vi "kinfe edge method.vi"(0 "Speed":cluster{"Speed":i32, "Vi":i32, "Vi steps":i32}={"Speed"=8000, "Vi"=1000, "Vi steps"=800} {"Speed" min=50 max=8000 step=50 scale=50.0..8000.0}, 1 "Go_stop":bool, 2 "PosCtrl":T5={"Go x"=FALSE, "Back x"=FALSE, "Go y"=FALSE, "Back y"=FALSE, "Go z"=FALSE, "Back z"=FALSE, "dX (um)"=1000, "dY (um)"=0, "dZ (um)"=0} {"dX (um)" step=1}, 5 "Home":bool, 7 "Zero":bool, 10 "stop 2":bool, 11 "VISA resource (RS232)":refnum<visa-resource-name>="COM1") -> (3 "?":cluster{"X":dbl, "Y":dbl, "Z":dbl}, 9 "Static":bool)   [LabVIEW 2018]
uses:
  <vilib>/userdefined/High Color/IMAQdx.ctl
  <vilib>/Instr/_visa.llb/VISA Configure Serial Port (Instr).vi
  <vilib>/vision/driver/NI_Vision_Acquisition_Software.lvlib
panel:
  out "t&Y error":dbl[][](array[numeric])
  out "um/s":string
  out "um(x) 2":string
  out "um(y)":string
  out "appended array":dbl[](array[numeric])
  out "fitting (y&T)":dbl[][](array[numeric])
  out "path (for logistic)":path
  out "row data save path":path
  in  "cluster":cluster{"T&Y(output)":dbl[][], "dt":dbl} {"dt" format="%#_13g"}
  out "T&Y(output)":dbl[][](array[numeric])
  out "Y(output)":dbl[](array[numeric])
  out "T(output)":dbl[](array[numeric])
  out "Initial X":dbl format="%^.3e"
  out "X Increment":dbl format="%^.3e"
  out "Y(all)":dbl[](array[numeric]) caption="Waveform Array" format="%^.3e"
  out "T(all)":dbl[](array[numeric])
  in  "Tout":i32
  in  "timeout":i32=5000 caption="Timeout\n[ms]"
  out "Waveform":T1(graph)
  out "Acquisitions":i32
  in  "Tab Control 2":enum32{"knife edge method", "Setting"}(tab)
  out "Snap Image":T2(plugin-control)
  in  "Get Image":bool
  in  "Tab Control":enum32{"Error function", "logistic function"}(tab)
  out "fitting":cluster{cdb[]}[](graph)
  in  "Paramter guess 2":dbl[](array[numeric])=[165.0, 0.2, 0.1]
  out "best fit parameters":dbl[](array[numeric])
  out "x0":dbl
  out "c":dbl
  in  "index":i32
  out "middle index(es)":i32
  out "number of function calls":i32
  in  "fitting(error)":bool caption="Fitting"
  in  "save(error)":bool caption="Fitting"
  in  "save(Logistic)":bool caption="Fitting"
  in  "fitting(Logistic)":bool caption="Fitting"
  out "output cluster 2":T3
  in  "Paramter guess":dbl[](array[numeric])=[-4.2, 0.0, 100.0, 1.0, 1.0]
  out "E":i32
  out "XY Graph":cluster{cdb[]}[](graph)
  out "output cluster":T4
  in  "speed(um/s)":i32
  in  "move(um)":i32
  in  "knife edge method":bool caption="Start"
  in  "knife edge method(stop)":bool caption="Start"
  in  "Tab Control 3":enum32{"read 2", "read", "cut & save"}(tab)
  in  "?":enum32{" RS232", "ESP32"}(tab)
  in  "x-":bool caption="Start"
  in  "x+":bool caption="Start"
  out "um(x)":string
  in  "y+":bool caption="Start"
  in  "y-":bool caption="Start"
  in  "um":i32
  in  "um":i32
  in  "channel on":i32=1 min=1 max=4 step=1
  out "ActiveChannels":i32[](array[numeric])=[1, 4]
  in  "Start":bool
  in  "Single":bool
  in  "Stop":bool
  in  "Exit":bool
  out "Samples count":i32[](array[numeric])
  out "waveform 3":cluster{"T":dbl[], "Waveform Array":dbl[]}(graph)
  out "point":i32
  in  "Path":path
  in  "name":string
  in  "Slide":cluster{dbl, dbl}(slide)={0.0, 1.2121212121212122} scale=0.10601..1.1059999999987864
  in  "Save data":bool caption="Fitting"
  out "waveform 2":cluster{"T":dbl[], "Waveform Array":dbl[]}(graph)
  out "Grab Image":T2(plugin-control)
  in  "?":bool
  in  "VISA resource name 2":refnum<visa-resource-name>="TCPIP0::169.254.236.131::inst0::INSTR" caption="VISA resource name"
  in  "VISA resource name":refnum<visa-resource-name>="TCPIP::169.254.236.131::HISLIP"
  out "Moving Time (Sec)":dbl
  in  "VISA resource (esp32)":refnum<visa-resource-name>="COM8"
  in  "Delay (ms)":u32=100
  in  "update period (ms)":u32=100
  in  "Go":bool
  in  "Back":bool
  in  "X0":T6 {"Y (um)" min=0.0; "X (um)" min=0.0}
  in  "Scaling":cluster{"X":u16, "Y":u16, "Z":u16} {"Z" items=["X", "Z", "None"]; "Y" items=["X", "Z", "None"]; "X" items=["X", "Z", "None"]}
  in  "Position to go":T7={"Position"={"X"=FALSE, "Target X (um)"=1000.0, "Current X (um)"=1000.0, "Scaling X"=0, "Y"=FALSE, "Target Y (um)"=0.0, "Current Y (um)"=0.0, "Scaling Y"=0, "Z"=FALSE, "Target Z (um)"=0.0, "Current Z (um)"=0.0, "Scaling Z"=0}, "Speed"={"Speed"=3111, "Vi steps"=800, "Vi"=1000}} {"Speed"."Speed" min=50 max=8000 step=50 scale=50.0..8000.0; "Position"."Current X (um)" step=1.0; "Position"."Scaling Z" items=["X", "Z", "None"]; "Position"."Scaling Y" items=["X", "Z", "None"]; "Position"."Scaling X" items=["X", "Z", "None"]; "Position"."Target X (um)" step=1.0}
  in  "Camera COM":T8
  out "Position Info":T9={"Current coordinates"={"Steps"=0.0, "X"=FALSE, "Steps 2"=0.0, "Y"=FALSE, "Steps 3"=0.0, "Z"=FALSE}, "read buffer"="", "Command"="a", "Current coordinates 2"={"X"=0.0, "Y"=0.0, "Z"=0.0}, "Moving Time (Sec)"=0.0}
  out "RS232 error":errorcluster
  # "Only For Knife Edge Method"
  # "y0\n\nx0\n\nK\n\nL\n\nA"
  # "Esp32"
  # "CCD"
  # "RTO"
  # "RS232"
  # "Origin"
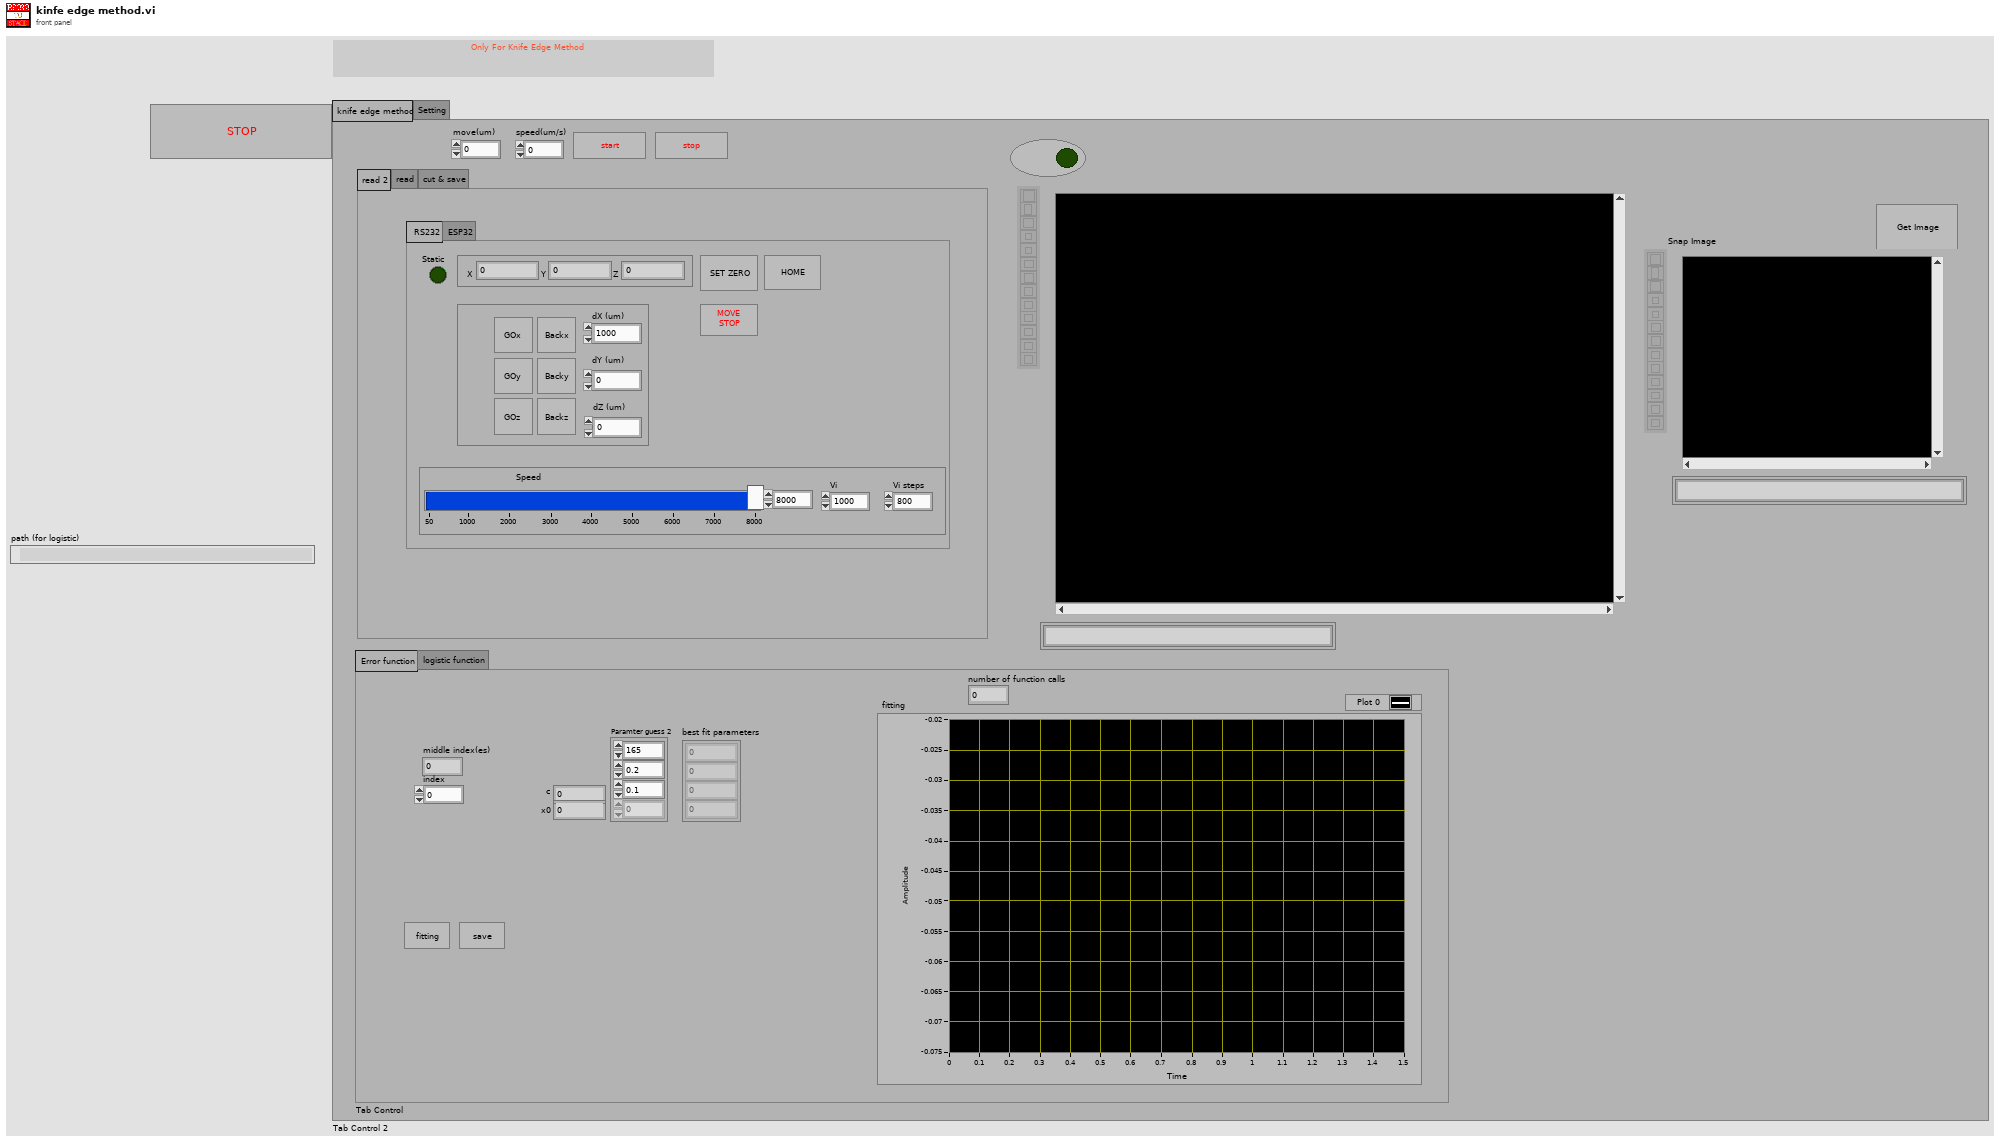
[diagram p1: front panel]
types:
  T1 = cluster{"Initial X":dbl, "X Increment":dbl, "Waveform Array":dbl[]}[]
  T2 = typedef "IMAQ Image.ctl" = refnum<image>
  T3 = cluster{"y0":dbl, "x0":dbl, "best fit parameters":dbl[]}
  T4 = cluster{"T(all)":dbl[], "Y(all)":dbl[], "X Increment":dbl, "Initial X":dbl}
  T5 = cluster{"Go x":bool, "Back x":bool, "Go y":bool, "Back y":bool, "Go z":bool, "Back z":bool, "dX (um)":u32, "dY (um)":u32, "dZ (um)":u32}
  T6 = cluster{"X (um)":dbl, "X 2":bool, "Y (um)":dbl, "Y 2":bool, "Z (um)":dbl, "Z 2":bool}
  T7 = cluster{"Position":cluster{"X":bool, "Target X (um)":dbl, "Current X (um)":dbl, "Scaling X":u16, "Y":bool, "Target Y (um)":dbl, "Current Y (um)":dbl, "Scaling Y":u16, "Z":bool, "Target Z (um)":dbl, "Current Z (um)":dbl, "Scaling Z":u16}, "Speed":cluster{"Speed":i32, "Vi steps":i32, "Vi":i32}}
  T8 = typedef "IMAQdx.ctl" = refnum<k21>
  T9 = cluster{"Current coordinates":cluster{"Steps":dbl, "X":bool, "Steps 2":dbl, "Y":bool, "Steps 3":dbl, "Z":bool}, "read buffer":string, "Command":string, "Current coordinates 2":cluster{"X":dbl, "Y":dbl, "Z":dbl}, "Moving Time (Sec)":dbl}
  T10 = cluster{"X":bool, "Target X (um)":dbl, "Current X (um)":dbl, "Scaling X":u16, "Y":bool, "Target Y (um)":dbl, "Current Y (um)":dbl, "Scaling Y":u16, "Z":bool, "Target Z (um)":dbl, "Current Z (um)":dbl, "Scaling Z":u16}
  T11 = cluster{"Go x":bool, "Back x":bool, "Go y":bool, "Back y":bool, "Go z":bool, "Back z":bool, "dX (um)":dbl, "dY (um)":dbl, "dZ (um)":dbl}
  T12 = cluster{"Position":cluster{"X":bool, "Target X (um)":dbl, "Current X (um)":dbl, "Scaling X":u16, "Y":bool, "Target Y (um)":dbl, "Current Y (um)":dbl, "Scaling Y":u16, "Z":bool, "Target Z (um)":dbl, "Current Z (um)":dbl, "Scaling Z":u16}, "Value":cluster{"Speed":i32, "Vi":i32, "Vi steps":i32}}
  T13 = cluster{"Task":u16, cluster{"Position":cluster{"X":bool, "Target X (um)":dbl, "Current X (um)":dbl, "Scaling X":u16, "Y":bool, "Target Y (um)":dbl, "Current Y (um)":dbl, "Scaling Y":u16, "Z":bool, "Target Z (um)":dbl, "Current Z (um)":dbl, "Scaling Z":u16}, "Value":cluster{"Speed":i32, "Vi":i32, "Vi steps":i32}}}
  T14 = cluster{"Task":u16, "Position to go":cluster{"Position":cluster{"X":bool, "Target X (um)":dbl, "Current X (um)":dbl, "Scaling X":u16, "Y":bool, "Target Y (um)":dbl, "Current Y (um)":dbl, "Scaling Y":u16, "Z":bool, "Target Z (um)":dbl, "Current Z (um)":dbl, "Scaling Z":u16}, "Speed":cluster{"Speed":i32, "Vi steps":i32, "Vi":i32}}}
  T15 = cluster{"Task 2":u16, "Position to go 2":cluster{"Position":cluster{"X":bool, "Target X (um)":dbl, "Current X (um)":dbl, "Scaling X":u16, "Y":bool, "Target Y (um)":dbl, "Current Y (um)":dbl, "Scaling Y":u16, "Z":bool, "Target Z (um)":dbl, "Current Z (um)":dbl, "Scaling Z":u16}, "Speed":cluster{"Speed":i32, "Vi steps":i32, "Vi":i32}}}
  T16 = cluster{"Go x":bool, "Back x":bool, "Go y":bool, "Back y":bool, "Go z":bool, "Back z":bool, "dX (um)":bool, "dY (um)":bool, "dZ (um)":bool}
  T17 = cluster{"Initial X":dbl, "X Increment":dbl, "Waveform Array":dbl[]}
  T18 = cluster{"Ring":u16, "Value":cluster{"Position":cluster{"X":bool, "Target X (um)":dbl, "Current X (um)":dbl, "Scaling X":u16, "Y":bool, "Target Y (um)":dbl, "Current Y (um)":dbl, "Scaling Y":u16, "Z":bool, "Target Z (um)":dbl, "Current Z (um)":dbl, "Scaling Z":u16}, "Speed":cluster{"Speed":i32, "Vi steps":i32, "Vi":i32}}}
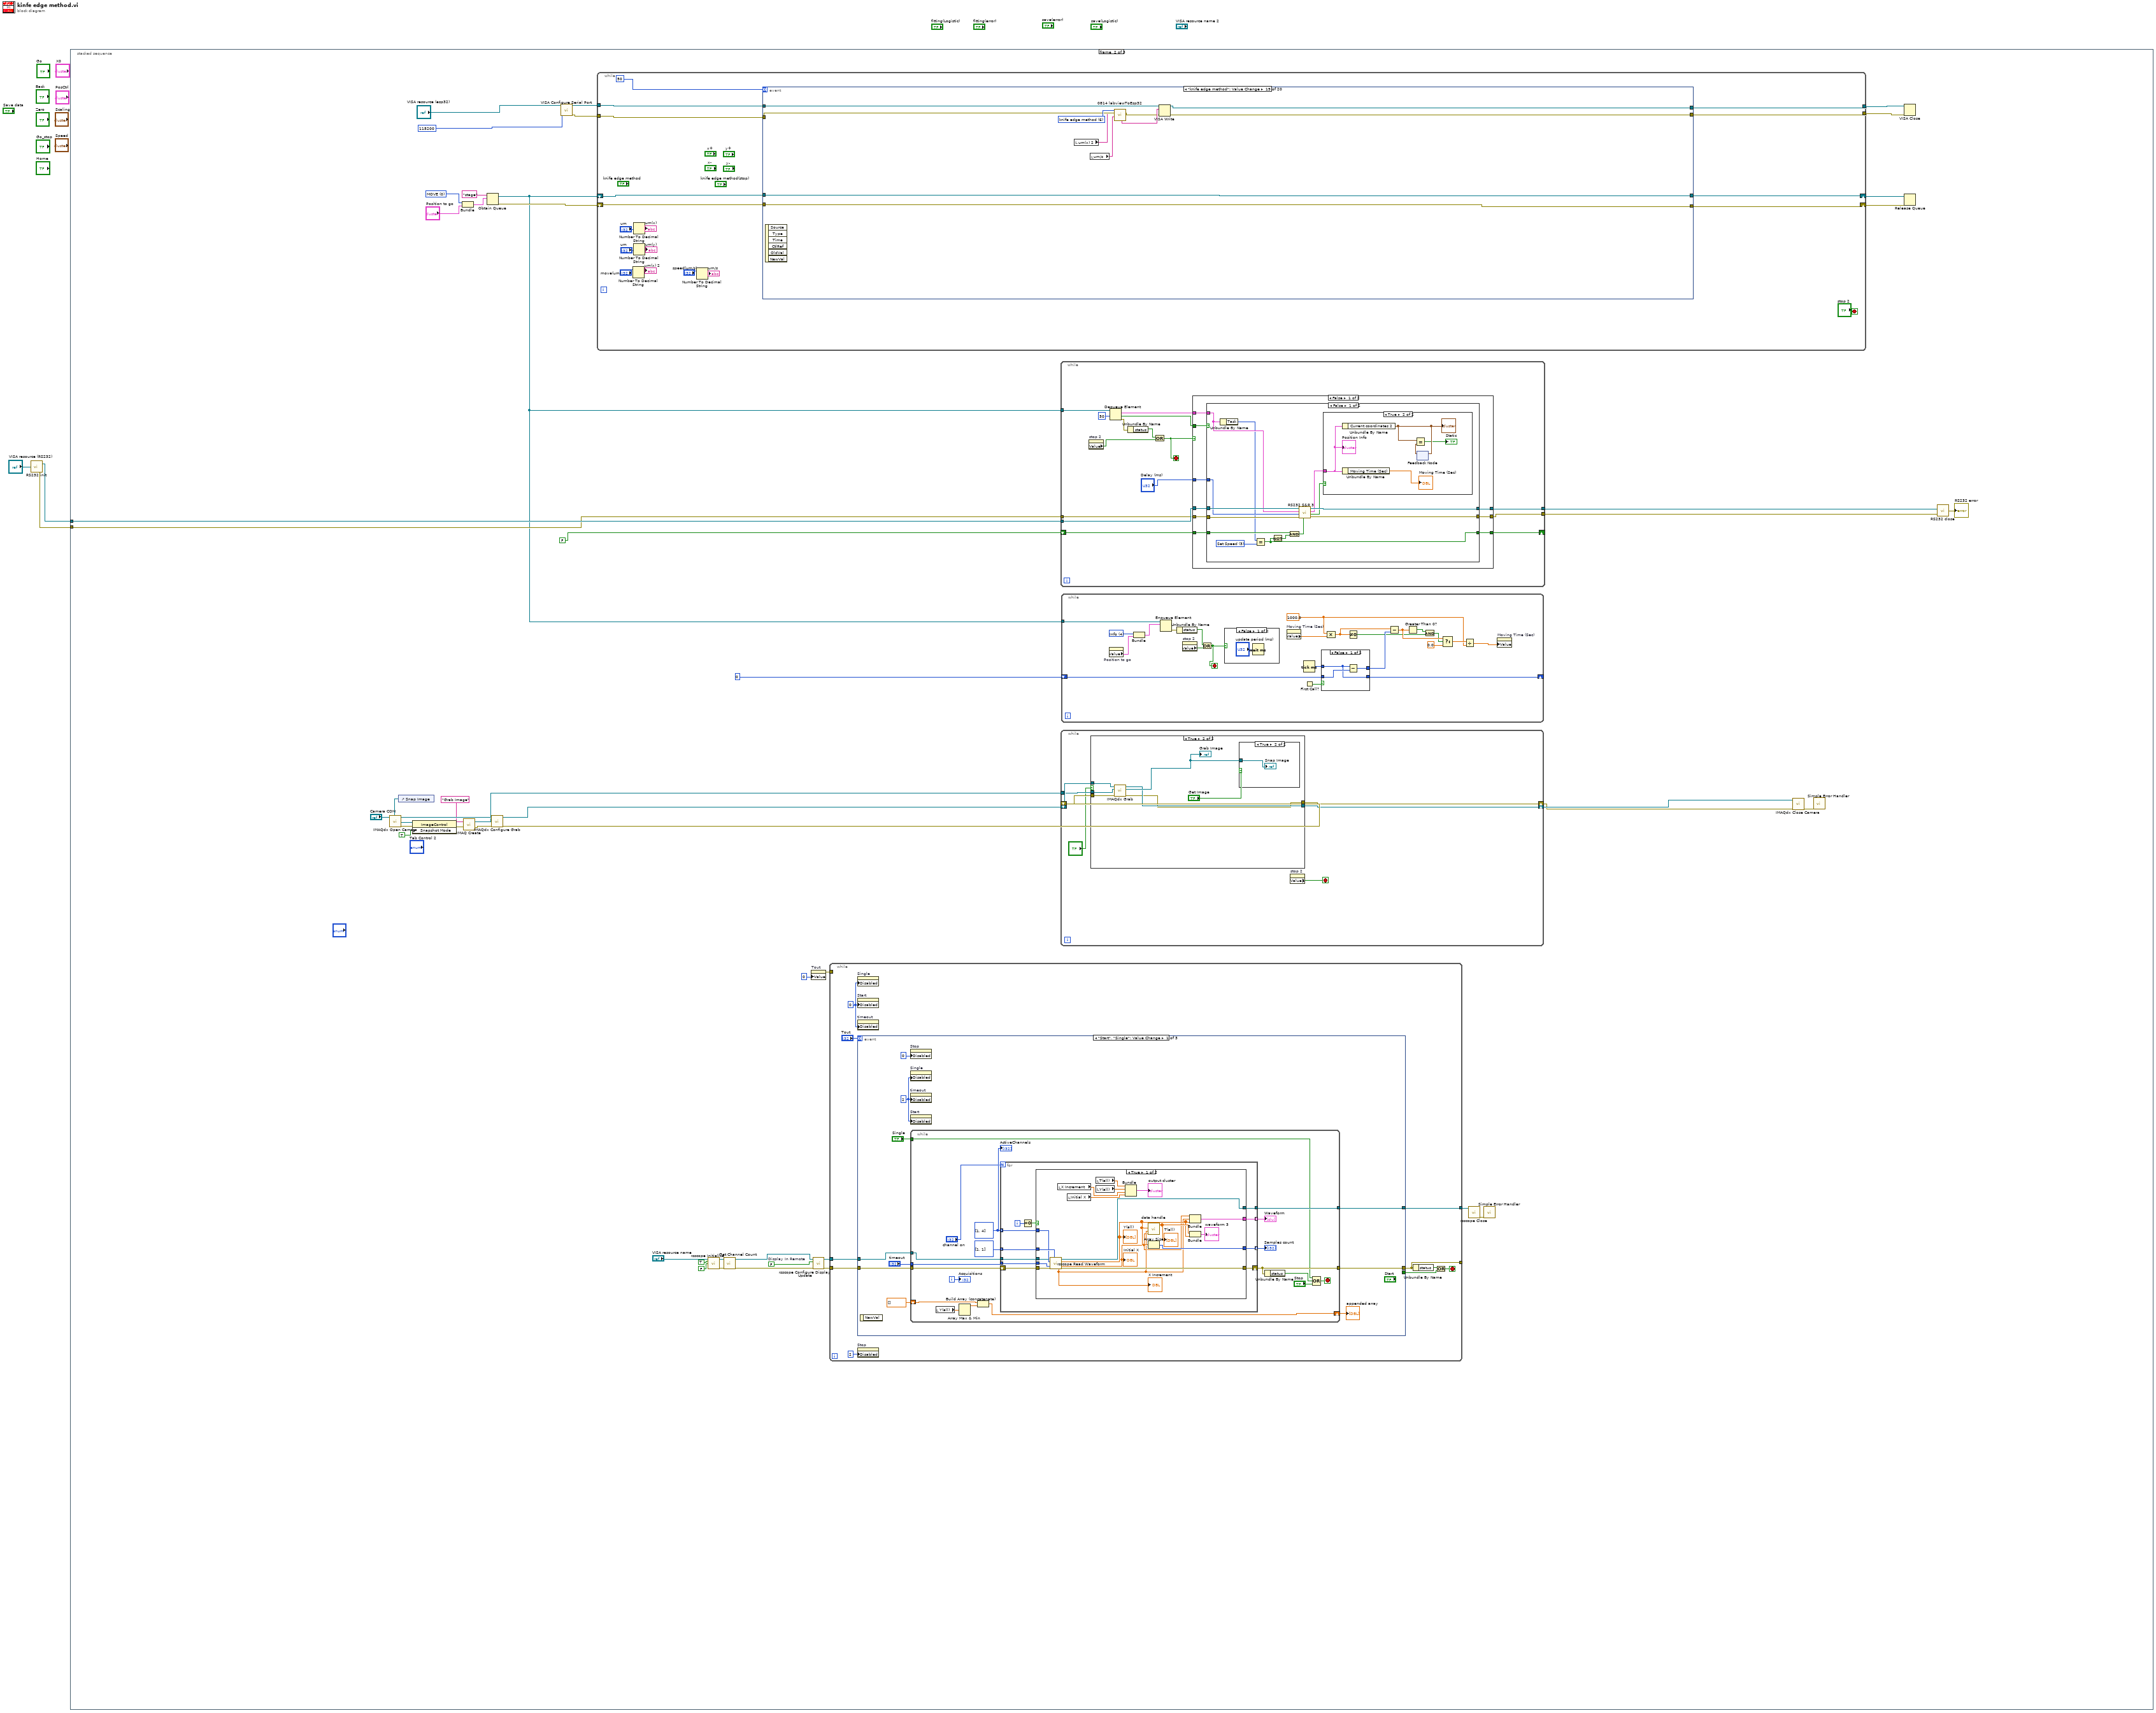
[diagram p0: block diagram]
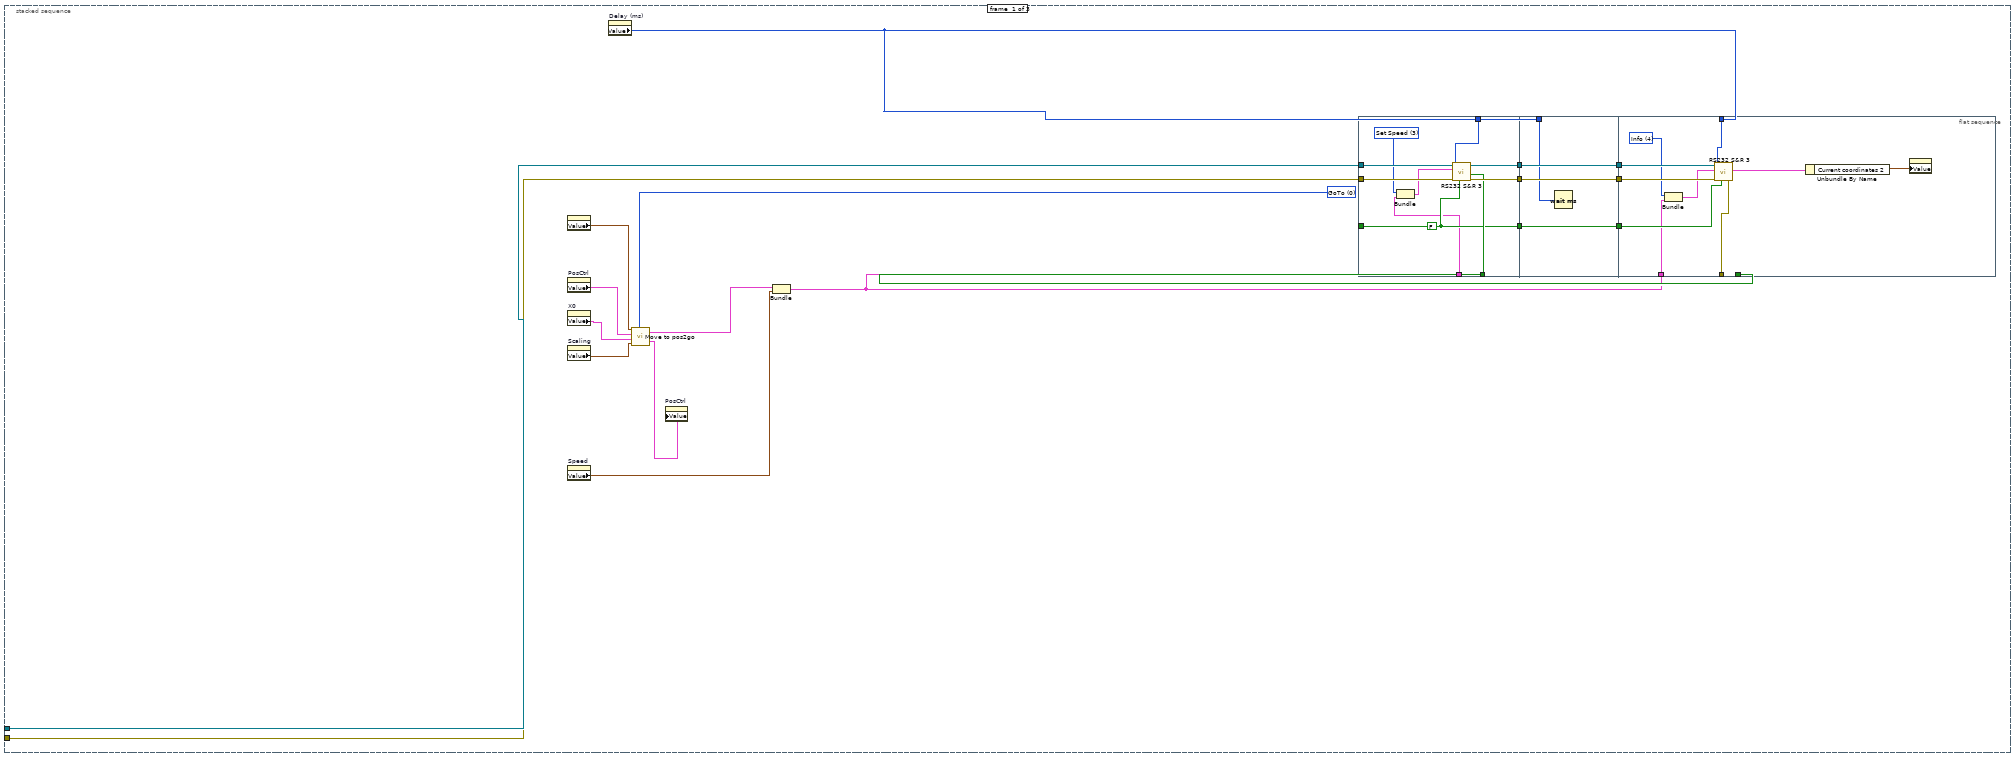
[diagram p2: hidden frame]
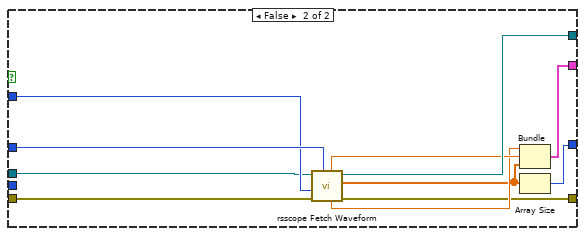
[diagram p3: hidden frame]
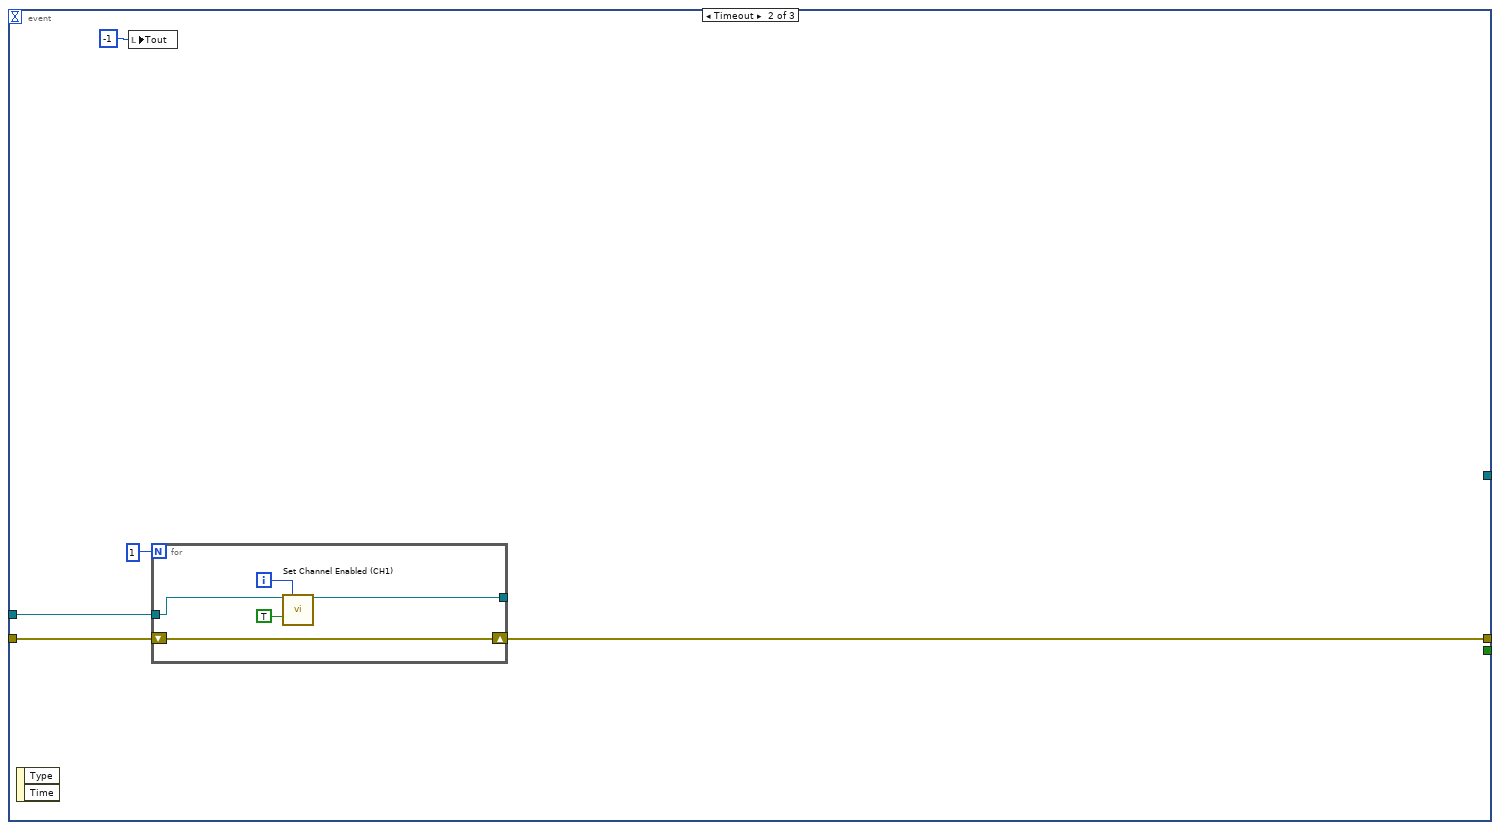
[diagram p4: hidden frame]
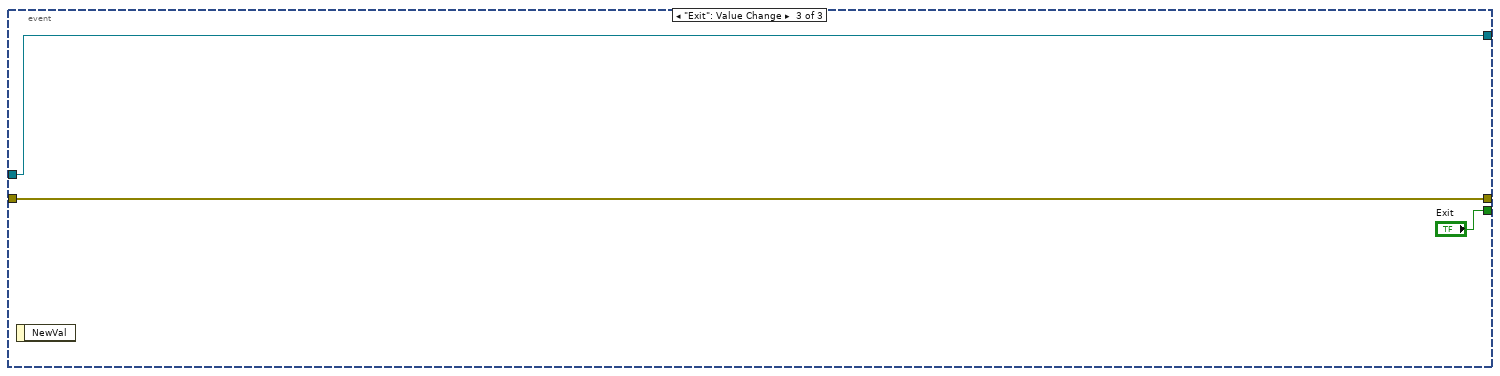
[diagram p5: hidden frame]
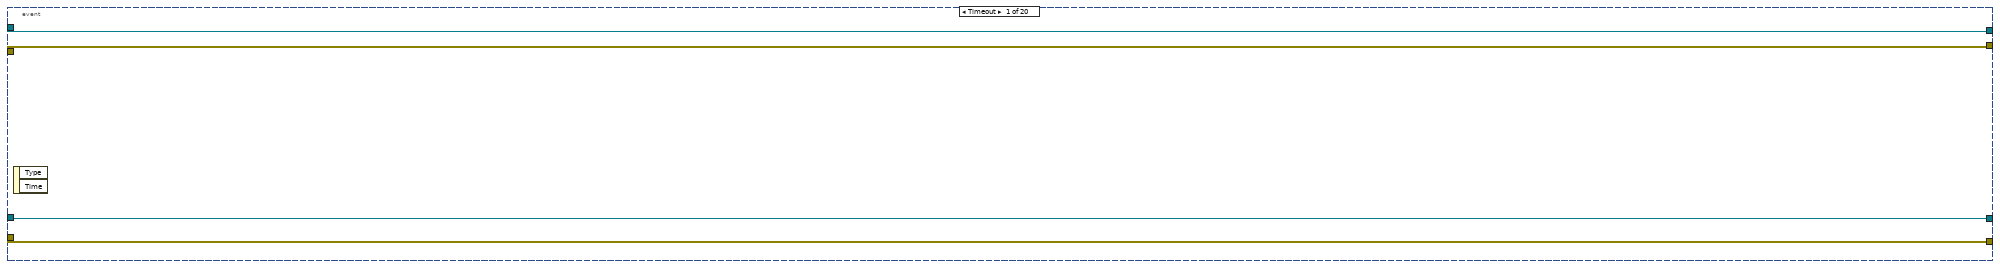
[diagram p13: hidden frame]
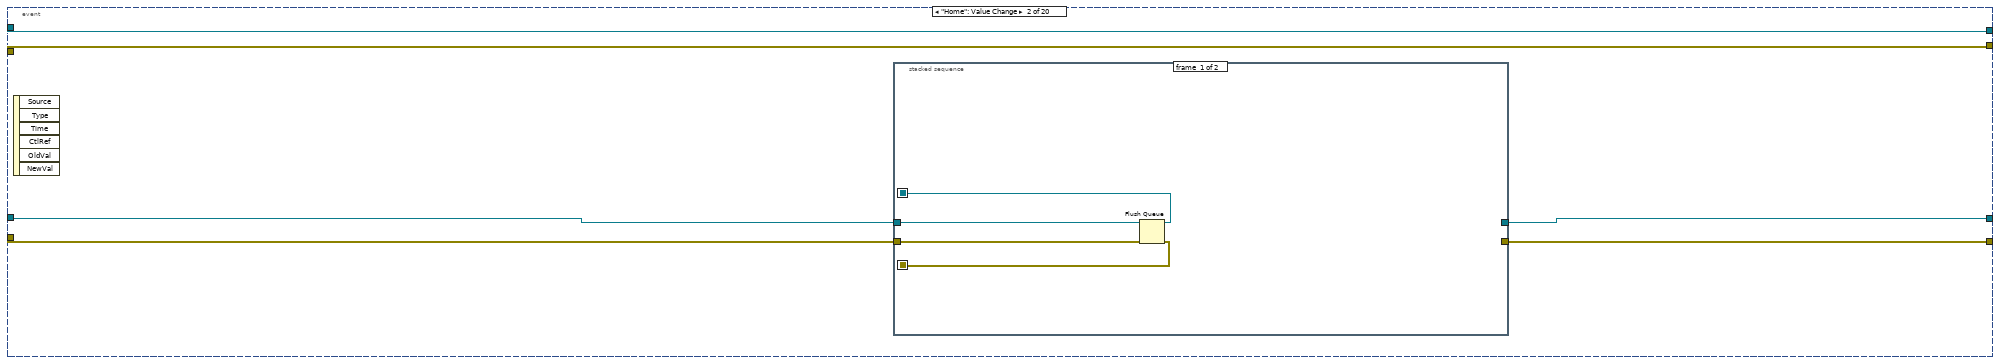
[diagram p14: hidden frame]
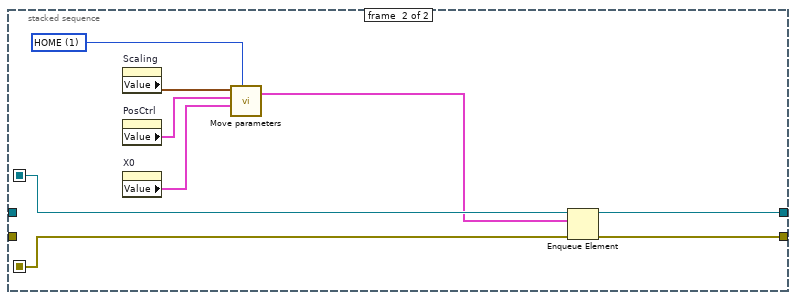
[diagram p15: hidden frame]
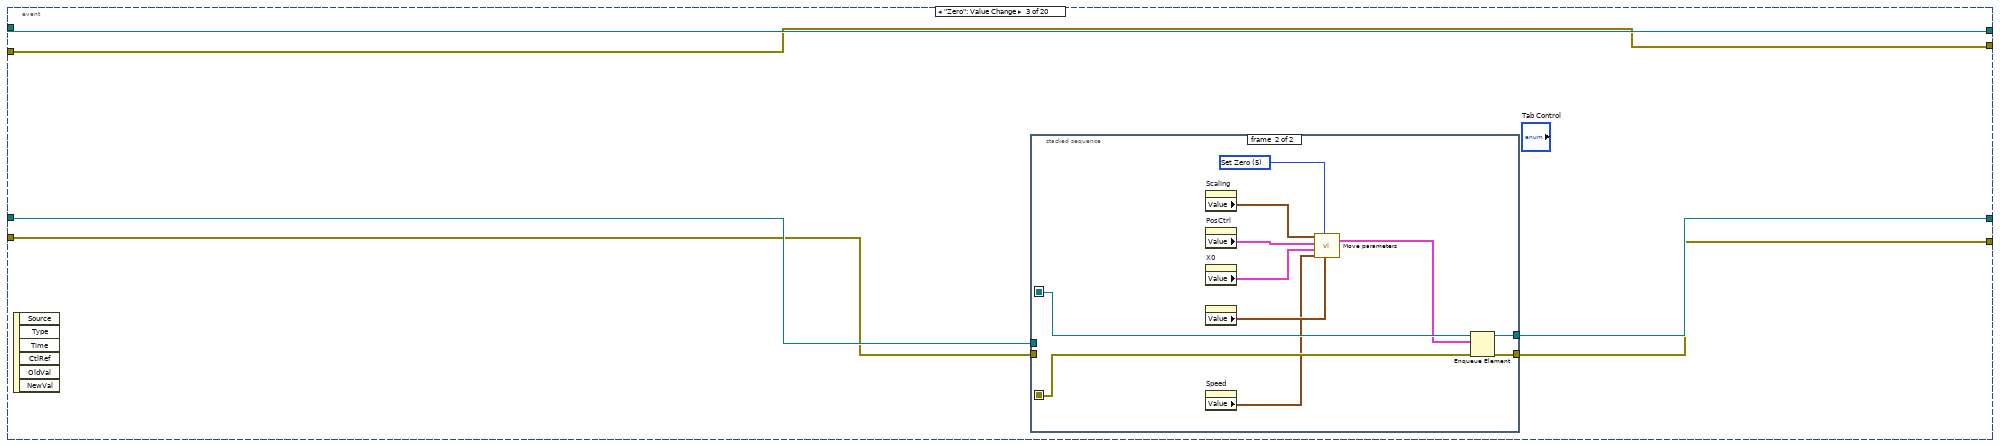
[diagram p16: hidden frame]
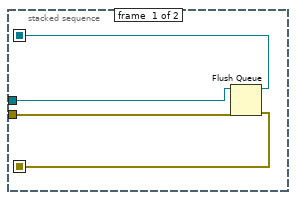
[diagram p17: hidden frame]
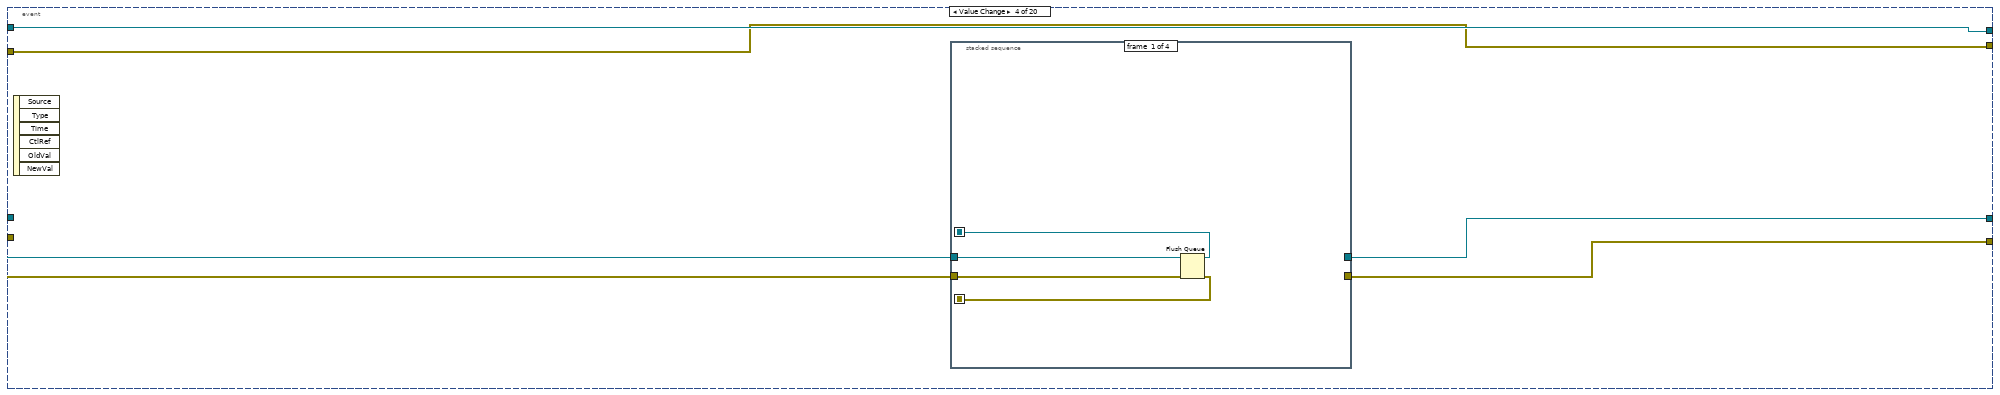
[diagram p18: hidden frame]
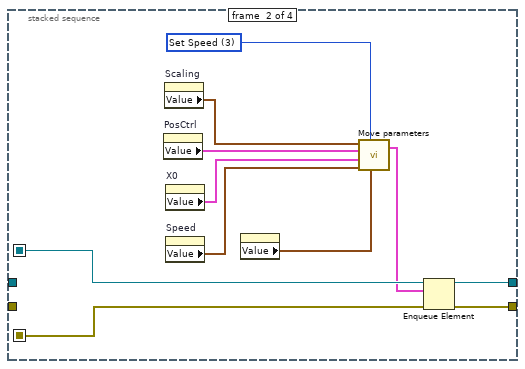
[diagram p19: hidden frame]
diagram:
  n1 = call "RS232 init.vi"("VISA resource name"="VISA resource (RS232)") -> ("VISA resource name out"=w2:refnum<visa-resource-name>, "error out"=w1:errorcluster)
  n2 = stacked-sequence {
    tunnel: w2 -> [w5 w89 _]
    tunnel: w1 -> [w4 w88 _]
    frame #0 {
      w10 = u16 0 items=["GoTo", "Jog"] ("Mode")
      n3 = property class="Clust (strict)"() -> ("Value"=w13:cluster{"X":dbl, "Y":dbl, "Z":dbl})  [unwired: 2 in, 2 out]
      n4 = property on="PosCtrl" class="Clust (strict)"() -> ("Value"=w12:T5)  [unwired: 2 in, 2 out]
      n5 = property on="X0" class="Clust (strict)"() -> ("Value"=w6:T6)  [unwired: 2 in, 2 out]
      n6 = property on="Scaling" class="Clust (strict)"() -> ("Value"=w11:cluster{"X":u16, "Y":u16, "Z":u16})  [unwired: 2 in, 2 out]
      n7 = property on="Speed" class="Clust (strict)"() -> ("Value"=w8:cluster{"Speed":i32, "Vi":i32, "Vi steps":i32})  [unwired: 2 in, 2 out]
      n8 = property on="Delay (ms)" class="DigNum (strict)"() -> ("Value"=w17:u32)  [unwired: 2 in, 2 out]
      n9 = call "Move to pos2go.vi"("Current coordinates"=w13, "DelX"=w12, "X0"=w6, "Scaling"=w11, "Mode"=w10) -> ("Position"=w9:T10, "DelX 2"=w7:T11)
      n10 = property on="PosCtrl" class="Clust (strict)"("Value"=w7) -> ()  [unwired: 2 in, 2 out]
      n11 = Bundle("Position"=w9, "Value"=w8) -> (w14:T12)  [unwired: 1 in]
      n12 = flat-sequence {
        tunnel: w5 -> [w33]
        tunnel: w4 -> [w32]
        tunnel: [w28] -> w15
        tunnel: w14 -> [w25]
        tunnel: [w31] -> w23
        tunnel: [w30] -> w22
        tunnel: w17 -> [w29]
        tunnel: FALSE -> [w27]
        tunnel: [w27] -> w21
        tunnel: [w37] -> w20
        tunnel: w23 -> [w37]
        tunnel: [w36] -> w19
        tunnel: w22 -> [w36]
        tunnel: w17 -> [w35]
        tunnel: [w34] -> w18
        tunnel: w21 -> [w34]
        tunnel: w20 -> [w47]
        tunnel: w19 -> [w46]
        tunnel: w17 -> [w45]
        tunnel: [w43] -> _
        tunnel: w15 -> [_]
        tunnel: w18 -> [w42]
        tunnel: w14 -> [w40]
        frame #0 {
          w26 = u16 3 items=["MOVE", "HOME", "STOP", "Set Speed", "Info", "Set Zero"] ("Task")
          n13 = Bundle("Task"=w26, w25) -> (w24:T13)  [unwired: 1 in]
          n14 = call "RS232 S&R 3.vi"("ReSetSPD"=w27, "error in"=w32, "Delay (ms)"=w29, "Stage Control"=w24, "VISA resource in"=w33) -> ("error out"=w30:errorcluster, "read"=w28:bool, "VISA resource name out"=w31:refnum<visa-resource-name>)  [unwired: 1 out]
        }
        frame #1 {
          n15 = Wait (ms)(milliseconds to wait=w35) -> ()  [unwired: 1 out]
        }
        frame #2 {
          w39 = u16 4 items=["MOVE", "HOME", "STOP", "Set Speed", "Info", "Set Zero"] ("Task")
          n16 = Bundle("Task"=w39, w40) -> (w38:T13)  [unwired: 1 in]
          n17 = call "RS232 S&R 3.vi"("ReSetSPD"=w42, "error in"=w46, "Delay (ms)"=w45, "Stage Control"=w38, "VISA resource in"=w47) -> ("error out"=w43:errorcluster, "Cluster"=w41:T9)  [unwired: 2 out]
          n18 = Unbundle By Name(w41) -> ("Current coordinates 2"=w44:cluster{"X":dbl, "Y":dbl, "Z":dbl})
          n19 = property class="Clust (strict)"("Value"=w44) -> ()  [unwired: 2 in, 2 out]
        }
      }
    }
    frame #1 {
      w54 = FALSE  # Display In Remote
      w94 = u16 0 items=["MOVE", "HOME", "STOP", "Set Speed", "Info", "Set Zero", "MOVE2"] ("Task")
      n20 = call <vilib>:"IMAQdx Open Camera.vi"("Session In"="Camera COM") -> ("error out"=w74:errorcluster, "Session Out"=w73:T8)  [unwired: 2 in, 7 out]
      n21 = control-ref of="Snap Image"() -> (w75:refnum<vi>)
      n22 = property class="ImageControl"(reference=w75, error in=w74, "Snapshot Mode"=TRUE) -> (error out=w72:errorcluster)  [unwired: 1 out]
      n23 = Bundle("Task"=w94, "Position to go"="Position to go") -> (w95:T14)  [unwired: 1 in]
      n24 = call "IMAQ Create"("Image Name"="Grab Image", "error in (no error)"=w72) -> ("New Image"=w62:T2, "error out"=w71:errorcluster)  [unwired: 2 in, 1 out]
      n25 = Obtain Queue(name (unnamed)="stage", element data type=w95) -> (queue out=w83:refnum<queue>, error out=w92:errorcluster)  [unwired: 3 in, 1 out]
      n26 = call <vilib>:"IMAQdx Configure Grab.vi"("error in"=w71, "Session In"=w73) -> ("error out"=w64:errorcluster, "Session Out"=w63:T8)  [unwired: 8 out]
      n27 = call-poly "VISA Configure Serial Port"("VISA resource name"="VISA resource (esp32)", "baud rate (9600)"=u32 115200) -> ("VISA resource name out"=w79:refnum<visa-resource-name>, "error out"=w78:errorcluster)  [unwired: 12 in]
      n28 = while {
        shift-right: [w299] -> w91
        shift-left: w83 -> [w302]
        shift-right: [w298] -> w90
        shift-left: w92 -> [w301]
        tunnel: w79 -> [w285]
        tunnel: w78 -> [w286]
        tunnel: [w297] -> w77
        tunnel: [w296] -> w76
        stop <- "stop 2" stop-if-true
        n29 = Number To Decimal String(number="move(um)") -> (decimal integer string=→"um(x) 2":string)  [unwired: 1 in]
        n30 = Number To Decimal String(number="um") -> (decimal integer string=→"um(x)":string)  [unwired: 1 in]
        n31 = Number To Decimal String(number="um") -> (decimal integer string=→"um(y)":string)  [unwired: 1 in]
        n32 = Number To Decimal String(number="speed(um/s)") -> (decimal integer string=→"um/s":string)  [unwired: 1 in]
        n33 = event shown="[18] \"knife edge method\": Value Change" {
          selector: _ -> [_ _ _ _ _ _ _ _ _ _ _ _ _ _ _ _ _ _ _ _]
          dyn-events: _ -> [_ _ _ _ _ _ _ _ _ _ _ _ _ _ _ _ _ _ _ _]
          timeout: 50 -> [_ _ _ _ _ _ _ _ _ _ _ _ _ _ _ _ _ _ _ _]
          tunnel: w302 -> [w306 w312 w331 w352 w373 w394 w415 w436 w479 w493 w501 w523 w527 w536 w543 w553 w563 w574 w587 w595]
          tunnel: w301 -> [w305 w311 w330 w351 w372 w393 w414 w435 w478 w492 w500 w522 w526 w535 w542 w552 w562 w573 w586 w594]
          tunnel: [w306 w310 w329 w350 w371 w392 w413 w434 w479 w493 w501 w523 w527 w536 w543 w553 w563 w574 w587 w595] -> w299
          tunnel: [w305 w309 w328 w349 w370 w391 w412 w433 w478 w492 w500 w522 w526 w535 w542 w552 w562 w573 w586 w594] -> w298
          tunnel: w285 -> [w304 w308 w327 w348 w369 w390 w411 w432 w481 w495 w503 w525 w529 w538 w547 w557 w567 w578 w589 w597]
          tunnel: w286 -> [w303 w307 w326 w347 w368 w389 w410 w431 w480 w494 w502 w524 w528 w537 w546 w556 w566 w577 w588 w596]
          tunnel: [w304 w308 w327 w348 w369 w390 w411 w432 w481 w495 w503 w525 w529 w538 w545 w555 w565 w576 w585 w593] -> w297
          tunnel: [w303 w307 w326 w347 w368 w389 w410 w431 w480 w494 w502 w524 w528 w537 w544 w554 w564 w575 w584 w592] -> w296
          event Timeout {
            n34 = event-data() -> ()  [unwired: 1 in, 2 out]
          }
          event "Home": Value Change {
            n35 = event-data() -> ()  [unwired: 1 in, 6 out]
            n36 = stacked-sequence {
              seq-local: [w313 _] -> [_ w323]
              seq-local: [w314 _] -> [_ w322]
              tunnel: w312 -> [w316 _]
              tunnel: w311 -> [w315 _]
              tunnel: [_ w325] -> w310
              tunnel: [_ w324] -> w309
              frame #0 {
                n37 = Flush Queue(queue=w316, error in (no error)=w315) -> (queue out=w313:refnum<queue>, error out=w314:errorcluster)  [unwired: 1 out]
              }
              frame #1 {
                w318 = u16 1 items=["MOVE", "HOME", "ZERO", "Set speed", "Info"] ("Ring")
                n38 = property on="Scaling" class="Clust (strict)"() -> ("Value"=w321:cluster{"X":u16, "Y":u16, "Z":u16})  [unwired: 2 in, 2 out]
                n39 = property on="PosCtrl" class="Clust (strict)"() -> ("Value"=w320:T5)  [unwired: 2 in, 2 out]
                n40 = property on="X0" class="Clust (strict)"() -> ("Value"=w317:T6)  [unwired: 2 in, 2 out]
                n41 = call "Move parameters.vi"("Task"=w318, "X0"=w317, "PosCtrl"=w320, "Scaling"=w321) -> ("Move info"=w319:T15)  [unwired: 2 in, 1 out]
                n42 = Enqueue Element(queue=w323, element=w319, error in (no error)=w322) -> (queue out=w325:refnum<queue>, error out=w324:errorcluster)  [unwired: 1 in, 1 out]
              }
            }
          }
          event "Zero": Value Change {
            n43 = event-data() -> ()  [unwired: 1 in, 6 out]
            n44 = stacked-sequence {
              seq-local: [w333 _] -> [_ w346]
              seq-local: [w334 _] -> [_ w345]
              tunnel: w330 -> [w335 _]
              tunnel: [_ w344] -> w329
              tunnel: [_ w343] -> w328
              tunnel: w331 -> [w332 _]
              frame #0 {
                n45 = Flush Queue(queue=w332, error in (no error)=w335) -> (queue out=w333:refnum<queue>, error out=w334:errorcluster)  [unwired: 1 out]
              }
              frame #1 {
                w342 = u16 5 items=["MOVE", "HOME", "STOP", "Set Speed", "Info", "Set Zero"] ("Task")
                n46 = property on="Scaling" class="Clust (strict)"() -> ("Value"=w340:cluster{"X":u16, "Y":u16, "Z":u16})  [unwired: 2 in, 2 out]
                n47 = property on="PosCtrl" class="Clust (strict)"() -> ("Value"=w339:T5)  [unwired: 2 in, 2 out]
                n48 = property on="X0" class="Clust (strict)"() -> ("Value"=w338:T6)  [unwired: 2 in, 2 out]
                n49 = property class="Clust (strict)"() -> ("Value"=w341:cluster{"X":dbl, "Y":dbl, "Z":dbl})  [unwired: 2 in, 2 out]
                n50 = property on="Speed" class="Clust (strict)"() -> ("Value"=w337:cluster{"Speed":i32, "Vi":i32, "Vi steps":i32})  [unwired: 2 in, 2 out]
                n51 = call "Move parameters.vi"("Current coordinates"=w341, "Task"=w342, "Speed"=w337, "X0"=w338, "PosCtrl"=w339, "Scaling"=w340) -> ("Move info"=w336:T15)  [unwired: 1 out]
                n52 = Enqueue Element(queue=w346, element=w336, error in (no error)=w345) -> (queue out=w344:refnum<queue>, error out=w343:errorcluster)  [unwired: 1 in, 1 out]
              }
            }
          }
          event "Speed.Speed": Value Change {
            n53 = event-data() -> ()  [unwired: 1 in, 6 out]
            n54 = stacked-sequence {
              seq-local: [w354 _ _ _] -> [_ w365 _ _]
              seq-local: [w353 _ _ _] -> [_ w364 _ _]
              tunnel: w352 -> [w356 _ _ _]
              tunnel: [_ w367 _ _] -> w350
              tunnel: w351 -> [w355 _ _ _]
              tunnel: [_ w366 _ _] -> w349
              frame #0 {
                n55 = Flush Queue(queue=w356, error in (no error)=w355) -> (queue out=w354:refnum<queue>, error out=w353:errorcluster)  [unwired: 1 out]
              }
              frame #1 {
                w363 = u16 3 items=["MOVE", "HOME", "STOP", "Set Speed", "Info", "Set Zero"] ("Task")
                n56 = property on="PosCtrl" class="Clust (strict)"() -> ("Value"=w361:T5)  [unwired: 2 in, 2 out]
                n57 = property on="Scaling" class="Clust (strict)"() -> ("Value"=w362:cluster{"X":u16, "Y":u16, "Z":u16})  [unwired: 2 in, 2 out]
                n58 = property on="X0" class="Clust (strict)"() -> ("Value"=w360:T6)  [unwired: 2 in, 2 out]
                n59 = property on="Speed" class="Clust (strict)"() -> ("Value"=w359:cluster{"Speed":i32, "Vi":i32, "Vi steps":i32})  [unwired: 2 in, 2 out]
                n60 = property class="Clust (strict)"() -> ("Value"=w358:cluster{"X":dbl, "Y":dbl, "Z":dbl})  [unwired: 2 in, 2 out]
                n61 = call "Move parameters.vi"("Current coordinates"=w358, "Task"=w363, "Speed"=w359, "X0"=w360, "PosCtrl"=w361, "Scaling"=w362) -> ("Move info"=w357:T15)  [unwired: 1 out]
                n62 = Enqueue Element(queue=w365, element=w357, error in (no error)=w364) -> (queue out=w367:refnum<queue>, error out=w366:errorcluster)  [unwired: 1 in, 1 out]
              }
              frame #2 {
              }
              frame #3 {
              }
            }
          }
          event "Go": Value Change {
            n63 = event-data() -> ()  [unwired: 1 in, 6 out]
            n64 = stacked-sequence {
              seq-local: [w374 _] -> [_ w386]
              seq-local: [w375 _] -> [_ w385]
              tunnel: w373 -> [w377 _]
              tunnel: w372 -> [w376 _]
              tunnel: [_ w388] -> w371
              tunnel: [_ w387] -> w370
              frame #0 {
                n65 = Flush Queue(queue=w377, error in (no error)=w376) -> (queue out=w374:refnum<queue>, error out=w375:errorcluster)  [unwired: 1 out]
              }
              frame #1 {
                w378 = u16 6 items=["MOVE", "HOME", "STOP", "Set Speed", "Info", "Set Zero", "MOVE2"] ("Task")
                n66 = property on="Scaling" class="Clust (strict)"() -> ("Value"=w382:cluster{"X":u16, "Y":u16, "Z":u16})  [unwired: 2 in, 2 out]
                n67 = property on="PosCtrl" class="Clust (strict)"() -> ("Value"=w383:T5)  [unwired: 2 in, 2 out]
                n68 = property on="X0" class="Clust (strict)"() -> ("Value"=w381:T6)  [unwired: 2 in, 2 out]
                n69 = property on="Speed" class="Clust (strict)"() -> ("Value"=w380:cluster{"Speed":i32, "Vi":i32, "Vi steps":i32})  [unwired: 2 in, 2 out]
                n70 = property class="Clust (strict)"() -> ("Value"=w379:cluster{"X":dbl, "Y":dbl, "Z":dbl})  [unwired: 2 in, 2 out]
                n71 = call "Move parameters.vi"("Current coordinates"=w379, "Task"=w378, "Speed"=w380, "X0"=w381, "PosCtrl"=w383, "Scaling"=w382) -> ("Move info"=w384:T15)  [unwired: 1 out]
                n72 = Enqueue Element(queue=w386, element=w384, error in (no error)=w385) -> (queue out=w388:refnum<queue>, error out=w387:errorcluster)  [unwired: 1 in, 1 out]
              }
            }
          }
          event "Back": Value Change {
            n73 = event-data() -> ()  [unwired: 1 in, 6 out]
            n74 = stacked-sequence {
              seq-local: [w395 _] -> [_ w407]
              seq-local: [w396 _] -> [_ w406]
              tunnel: w394 -> [w398 _]
              tunnel: w393 -> [w397 _]
              tunnel: [_ w409] -> w392
              tunnel: [_ w408] -> w391
              frame #0 {
                n75 = Flush Queue(queue=w398, error in (no error)=w397) -> (queue out=w395:refnum<queue>, error out=w396:errorcluster)  [unwired: 1 out]
              }
              frame #1 {
                w399 = u16 6 items=["MOVE", "HOME", "STOP", "Set Speed", "Info", "Set Zero", "MOVE2"] ("Task")
                n76 = property on="Scaling" class="Clust (strict)"() -> ("Value"=w403:cluster{"X":u16, "Y":u16, "Z":u16})  [unwired: 2 in, 2 out]
                n77 = property on="PosCtrl" class="Clust (strict)"() -> ("Value"=w404:T5)  [unwired: 2 in, 2 out]
                n78 = property on="X0" class="Clust (strict)"() -> ("Value"=w402:T6)  [unwired: 2 in, 2 out]
                n79 = property on="Speed" class="Clust (strict)"() -> ("Value"=w401:cluster{"Speed":i32, "Vi":i32, "Vi steps":i32})  [unwired: 2 in, 2 out]
                n80 = property class="Clust (strict)"() -> ("Value"=w400:cluster{"X":dbl, "Y":dbl, "Z":dbl})  [unwired: 2 in, 2 out]
                n81 = call "Move parameters.vi"("Current coordinates"=w400, "Task"=w399, "Speed"=w401, "X0"=w402, "PosCtrl"=w404, "Scaling"=w403) -> ("Move info"=w405:T15)  [unwired: 1 out]
                n82 = Enqueue Element(queue=w407, element=w405, error in (no error)=w406) -> (queue out=w409:refnum<queue>, error out=w408:errorcluster)  [unwired: 1 in, 1 out]
              }
            }
          }
          event "Go_stop": Value Change {
            n83 = event-data() -> ()  [unwired: 1 in, 6 out]
            n84 = stacked-sequence {
              seq-local: [w416 _] -> [_ w427]
              seq-local: [w417 _] -> [_ w428]
              tunnel: w415 -> [w419 _]
              tunnel: w414 -> [w418 _]
              tunnel: [_ w430] -> w413
              tunnel: [_ w429] -> w412
              frame #0 {
                n85 = Flush Queue(queue=w419, error in (no error)=w418) -> (queue out=w416:refnum<queue>, error out=w417:errorcluster)  [unwired: 1 out]
              }
              frame #1 {
                w426 = u16 2 items=["MOVE", "HOME", "STOP", "Set Speed", "Info", "Set Zero"] ("Task")
                n86 = property on="Scaling" class="Clust (strict)"() -> ("Value"=w425:cluster{"X":u16, "Y":u16, "Z":u16})  [unwired: 2 in, 2 out]
                n87 = property on="PosCtrl" class="Clust (strict)"() -> ("Value"=w424:T5)  [unwired: 2 in, 2 out]
                n88 = property on="X0" class="Clust (strict)"() -> ("Value"=w423:T6)  [unwired: 2 in, 2 out]
                n89 = property on="Speed" class="Clust (strict)"() -> ("Value"=w422:cluster{"Speed":i32, "Vi":i32, "Vi steps":i32})  [unwired: 2 in, 2 out]
                n90 = property class="Clust (strict)"() -> ("Value"=w421:cluster{"X":dbl, "Y":dbl, "Z":dbl})  [unwired: 2 in, 2 out]
                n91 = call "Move parameters.vi"("Current coordinates"=w421, "Task"=w426, "Speed"=w422, "X0"=w423, "PosCtrl"=w424, "Scaling"=w425) -> ("Move info"=w420:T15)  [unwired: 1 out]
                n92 = Enqueue Element(queue=w427, element=w420, error in (no error)=w428) -> (queue out=w430:refnum<queue>, error out=w429:errorcluster)  [unwired: 1 in, 1 out]
              }
            }
          }
          event "PosCtrl": Value Change {
            n93 = event-data() -> ("OldVal"=w439:T5, "NewVal"=w438:T5)  [unwired: 1 in, 4 out]
            n94 = Equal?(x=w439, y=w438) -> (x = y?=w446:T16)
            n95 = Unbundle By Name(w446) -> ("Go x"=w445:bool, "Back x"=w444:bool, "Go y"=w443:bool, "Back y"=w442:bool, "Go z"=w441:bool, "Back z"=w440:bool)
            n96 = Compound Arithmetic op=OR(w445, w444, w443, w442, w441, w440) -> (w437:bool)
            n97 = case shown="True" w437 {
              tunnel: [w448 w452] -> w434
              tunnel: [w447 w451] -> w433
              tunnel: w436 -> [w448 w450]
              tunnel: w435 -> [w447 w449]
              frame False {
              }
              frame True {
                n98 = stacked-sequence {
                  seq-local: [w453 _ _] -> [_ w465 _]
                  seq-local: [w454 _ _] -> [_ w466 _]
                  seq-local: [_ w457 _] -> [_ _ w469]
                  tunnel: w450 -> [w456 _ _]
                  tunnel: w449 -> [w455 _ _]
                  tunnel: [_ w468 _] -> w452
                  tunnel: [_ w467 _] -> w451
                  frame #0 {
                    n99 = Flush Queue(queue=w456, error in (no error)=w455) -> (queue out=w453:refnum<queue>, error out=w454:errorcluster)  [unwired: 1 out]
                  }
                  frame #1 {
                    w458 = u16 0 items=["MOVE", "HOME", "STOP", "Set Speed", "Info", "Set Zero", "MOVE2"] ("Task")
                    n100 = property on="Scaling" class="Clust (strict)"() -> ("Value"=w464:cluster{"X":u16, "Y":u16, "Z":u16})  [unwired: 2 in, 2 out]
                    n101 = property on="PosCtrl" class="Clust (strict)"() -> ("Value"=w463:T5)  [unwired: 2 in, 2 out]
                    n102 = property on="X0" class="Clust (strict)"() -> ("Value"=w462:T6)  [unwired: 2 in, 2 out]
                    n103 = property on="Speed" class="Clust (strict)"() -> ("Value"=w461:cluster{"Speed":i32, "Vi":i32, "Vi steps":i32})  [unwired: 2 in, 2 out]
                    n104 = property class="Clust (strict)"() -> ("Value"=w460:cluster{"X":dbl, "Y":dbl, "Z":dbl})  [unwired: 2 in, 2 out]
                    n105 = call "Move parameters.vi"("Current coordinates"=w460, "Task"=w458, "Speed"=w461, "X0"=w462, "PosCtrl"=w463, "Scaling"=w464) -> ("PosCtrl out"=w457:T11, "Move info"=w459:T15)
                    n106 = Enqueue Element(queue=w465, element=w459, error in (no error)=w466) -> (queue out=w468:refnum<queue>, error out=w467:errorcluster)  [unwired: 1 in, 1 out]
                  }
                  frame #2 {
                    n107 = property on="PosCtrl" class="Clust (strict)"("Value"=w469) -> ()  [unwired: 2 in, 2 out]
                  }
                }
              }
            }
          }
          event "Slide": Value Change {
            n108 = event-data() -> ()  [unwired: 1 in, 6 out]
            n109 = local read "T&Y(output)"() -> (w473:dbl[][])
            n110 = local read "X Increment"() -> (w475:dbl)
            n111 = Transpose 2D Array(2D array=w473) -> (transposed array=w472:dbl[][])
            n112 = Bundle(w472, "X Increment"=w475) -> (w474:cluster{dbl[][], "X Increment":dbl})  [unwired: 1 in]
            n113 = local read "output cluster"() -> (w490:T4)
            n114 = local write "cluster"(w474) -> ()
            n115 = Unbundle(w490) -> ("T(all)"=w489:dbl[], "Y(all)"=w488:dbl[], "X Increment"=w486:dbl, "Initial X"=w487:dbl)
            n116 = call "split data.vi"("Slide"="Slide", "dt"=w486, "t0"=w487, "Y(input)"=w488, "T(input)"=w489) -> ("max value"=w483:dbl, "min value"=w484:dbl, "Y(output)"=w471:dbl[], "T(output)"=w477:dbl[])  [unwired: 2 in]
            "T(output)" <- w477
            "Y(output)" <- w471
            n117 = property on="Slide" class="Slide (strict)"("Scale.Maximum"=w483, "Scale.Minimum"=w484) -> ()  [unwired: 2 in, 2 out]
            n118 = Bundle("T(output)"=w477, "Y(output)"=w471) -> (→"waveform 2":cluster{"T(output)":dbl[], "Y(output)":dbl[]})  [unwired: 1 in]
            n119 = Array Size(array=w471) -> (size(s)=→"point":i32)
            n120 = Build Array(w477, w471) -> (→"T&Y(output)":dbl[][])
          }
          event "Save data": Value Change {
            n121 = event-data() -> ()  [unwired: 1 in, 6 out]
            n122 = call "save data.vi"("name"="name", "Path"="Path", "cluster"="cluster") -> ("new file path (Not A Path if cancelled)"=→"row data save path":path, "path(FOR logistic"=→"path (for logistic)":path)  [unwired: 6 in, 1 out]
          }
          event "fitting(Logistic)": Value Change {
            n123 = event-data() -> ()  [unwired: 1 in, 6 out]
            n124 = local read "Y(output)"() -> (w509:dbl[])
            n125 = local read "T(output)"() -> (w510:dbl[])
            n126 = call "Fittinglogistic_MODCA.vi"("Paramter guess"="Paramter guess", "y"=w509, "t"=w510) -> ("fitting (y&T)"=→"fitting (y&T)":dbl[][], "E"=→"E":i32, "XY Graph"=→"XY Graph":cluster{cdb[]}[], "output cluster"=→"output cluster 2":T3)  [unwired: 5 in]
          }
          event "fitting(error)": Value Change {
            n127 = event-data() -> ()  [unwired: 1 in, 6 out]
            n128 = local read "Y(output)"() -> (w520:dbl[])
            n129 = local read "T(output)"() -> (w521:dbl[])
            n130 = call "FittingGaussianKnife_MODCA.vi"("Paramter guess"="Paramter guess 2", "index"="index", "y(in)"=w520, "x(in)"=w521) -> ("number of function calls"=→"number of function calls":i32, "fitting"=→"fitting":cluster{cdb[]}[], "best fit parameters"=→"best fit parameters":dbl[], "x0"=→"x0":dbl, "t&Y error"=→"t&Y error":dbl[][], "c"=→"c":dbl, "middle index(es)"=→"middle index(es)":i32)  [unwired: 1 out]
          }
          event "save(Logistic)": Value Change {
            n131 = event-data() -> ()  [unwired: 1 in, 6 out]
            n132 = local read "path (for logistic)"() -> (w530:path)
            n133 = local read "fitting (y&T)"() -> (w531:dbl[][])
            n134 = local read "Paramter guess"() -> (w533:dbl[])
            n135 = call "error save.vi"("file path (dialog if empty)"=w530, "format (%.3f)"="%.7e", "Paramter guess"=w533, "2D data"=w531) -> ()  [unwired: 10 in, 2 out]
          }
          event "save(error)": Value Change {
            n136 = event-data() -> ()  [unwired: 1 in, 6 out]
            n137 = local read "path (for logistic)"() -> (w539:path)
            n138 = local read "t&Y error"() -> (w534:dbl[][])
            n139 = local read "Paramter guess 2"() -> (w541:dbl[])
            n140 = call "error save.vi"("file path (dialog if empty)"=w539, "format (%.3f)"="%.7e", "Paramter guess"=w541, "2D data"=w534) -> ()  [unwired: 10 in, 2 out]
          }
          event "x+": Value Change {
            w551 = u16 1 items=["Move X"=1, "Move Y"=2, "Single shot"=3, "single shot *15"=4, "energy adjustment"=5, "knife edge method"=6, "Auto mode"=7] ("Ring")
            n141 = event-data() -> ()  [unwired: 1 in, 6 out]
            n142 = local read "um(x)"() -> (w549:string)
            n143 = call "0814 labviewToEsp32.vi"("direction"="0", "um"=w549, "Ring"=w551) -> ("output"=w548:string)  [unwired: 8 in]
            n144 = VISA Write(VISA resource name=w547, write buffer=w548, error in (no error)=w546) -> (VISA resource name out=w545:refnum<visa-resource-name>, error out=w544:errorcluster)  [unwired: 1 out]
          }
          event "x-": Value Change {
            w561 = u16 1 items=["Move X"=1, "Move Y"=2, "Single shot"=3, "single shot *15"=4, "energy adjustment"=5, "knife edge method"=6, "Auto mode"=7] ("Ring")
            n145 = event-data() -> ()  [unwired: 1 in, 6 out]
            n146 = local read "um(x)"() -> (w559:string)
            n147 = call "0814 labviewToEsp32.vi"("direction"="1", "um"=w559, "Ring"=w561) -> ("output"=w558:string)  [unwired: 8 in]
            n148 = VISA Write(VISA resource name=w557, write buffer=w558, error in (no error)=w556) -> (VISA resource name out=w555:refnum<visa-resource-name>, error out=w554:errorcluster)  [unwired: 1 out]
          }
          event "y+": Value Change {
            w571 = u16 2 items=["Move X"=1, "Move Y"=2, "Single shot"=3, "single shot *15"=4, "energy adjustment"=5, "knife edge method"=6, "Auto mode"=7] ("Ring")
            n149 = event-data() -> ()  [unwired: 1 in, 6 out]
            n150 = local read "um(y)"() -> (w568:string)
            n151 = call "0814 labviewToEsp32.vi"("direction"="0", "um"=w568, "Ring"=w571) -> ("output"=w569:string)  [unwired: 8 in]
            n152 = VISA Write(VISA resource name=w567, write buffer=w569, error in (no error)=w566) -> (VISA resource name out=w565:refnum<visa-resource-name>, error out=w564:errorcluster)  [unwired: 1 out]
          }
          event "y-": Value Change {
            w581 = u16 2 items=["Move X"=1, "Move Y"=2, "Single shot"=3, "single shot *15"=4, "energy adjustment"=5, "knife edge method"=6, "Auto mode"=7] ("Ring")
            n153 = event-data() -> ()  [unwired: 1 in, 6 out]
            n154 = local read "um(y)"() -> (w572:string)
            n155 = call "0814 labviewToEsp32.vi"("direction"="1", "um"=w572, "Ring"=w581) -> ("output"=w579:string)  [unwired: 8 in]
            n156 = VISA Write(VISA resource name=w578, write buffer=w579, error in (no error)=w577) -> (VISA resource name out=w576:refnum<visa-resource-name>, error out=w575:errorcluster)  [unwired: 1 out]
          }
          event "knife edge method": Value Change {
            w591 = u16 6 items=["Move X"=1, "Move Y"=2, "Single shot"=3, "single shot *15"=4, "energy adjustment"=5, "knife edge method"=6, "Auto mode"=7] ("Ring")
            n157 = event-data() -> ()  [unwired: 1 in, 6 out]
            n158 = local read "um(x) 2"() -> (w582:string)
            n159 = local read "um/s"() -> (w583:string)
            n160 = call "0814 labviewToEsp32.vi"("count"=w583, "um"=w582, "Ring"=w591) -> ("output"=w590:string)  [unwired: 8 in]
            n161 = VISA Write(VISA resource name=w589, write buffer=w590, error in (no error)=w588) -> (VISA resource name out=w585:refnum<visa-resource-name>, error out=w584:errorcluster)  [unwired: 1 out]
          }
          event "knife edge method(stop)": Value Change {
            w599 = u16 0 items=["Move X"=1, "Move Y"=2, "Single shot"=3, "single shot *15"=4, "energy adjustment"=5, "knife edge method"=6, "Auto mode"=7, "multiple shot"=8, "stop"=0] ("Ring")
            n162 = event-data() -> ()  [unwired: 1 in, 6 out]
            n163 = call "0814 labviewToEsp32.vi"("Ring"=w599) -> ("output"=w598:string)  [unwired: 10 in]
            n164 = VISA Write(VISA resource name=w597, write buffer=w598, error in (no error)=w596) -> (VISA resource name out=w593:refnum<visa-resource-name>, error out=w592:errorcluster)  [unwired: 1 out]
          }
        }
      }
      n165 = call "rsscope Initialize.vi"("VISA resource name"="VISA resource name", "ID Query (T: Check)"=TRUE, "Reset (T: Reset)"=FALSE) -> ("VISA resource name out"=w56:refnum<visa-resource-name>, "error out"=w57:errorcluster)  [unwired: 11 in]
      n166 = call "Get Channel Count"("instrument handle"=w56, "error in (no error)"=w57) -> ("instrument handle out"=w55:refnum<visa-resource-name>, "error out"=w50:errorcluster)  [unwired: 11 in, 1 out]
      n167 = property on="Tout" class="DigNum (strict)"("Value"=0 ("Tout")) -> (error out=w60:errorcluster)  [unwired: 2 in, 1 out]
      n168 = call "rsscope Configure Display Update.vi"("error in (no error)"=w50, "Display In Remote (Off)"=w54, "VISA resource name"=w55) -> ("error out"=w53:errorcluster, "VISA resource name out"=w52:refnum<visa-resource-name>)  [unwired: 7 in]
      n169 = while {
        tunnel: w60 -> [_]
        tunnel: [w99] -> _
        tunnel: w53 -> [w102]
        tunnel: w52 -> [w101]
        tunnel: [w100] -> w51
        stop <- w106 stop-if-true
        w103 = u8 0 ("Disabled")
        n170 = property on="Single" class="Bool"("Disabled"=w103) -> ()  [unwired: 2 in, 2 out]
        n171 = property on="Start" class="Bool"("Disabled"=w103) -> ()  [unwired: 2 in, 2 out]
        n172 = property on="timeout" class="DigNum (strict)"("Disabled"=w103) -> ()  [unwired: 2 in, 2 out]
        n173 = event shown="[0] \"Start\", \"Single\": Value Change" {
          selector: _ -> [_ _ _]
          dyn-events: _ -> [_ _ _]
          timeout: "Tout" -> [_ _ _]
          tunnel: [w116 _ w187] -> w100
          tunnel: w102 -> [w110 w179 w188]
          tunnel: [w115 w181 w188] -> w99
          tunnel: w101 -> [w111 w178 w187]
          tunnel: [_ _ "Exit"] -> w97
          event "Start", "Single": Value Change {
            w112 = u8 2 ("Disabled")
            n174 = event-data() -> ()  [unwired: 1 in, 1 out]
            n175 = property on="Stop" class="Bool"("Disabled"=u8 0) -> ()  [unwired: 2 in, 2 out]
            n176 = property on="Single" class="Bool"("Disabled"=w112) -> ()  [unwired: 2 in, 2 out]
            n177 = property on="timeout" class="DigNum (strict)"("Disabled"=w112) -> ()  [unwired: 2 in, 2 out]
            n178 = property on="Start" class="Bool"("Disabled"=w112) -> ()  [unwired: 2 in, 2 out]
            n179 = while {
              tunnel: "timeout" -> [w135]
              tunnel: [w133] -> w115
              tunnel: [w134] -> w116
              tunnel: w111 -> [w127]
              tunnel: w110 -> [w126]
              tunnel: "Single" -> [w125]
              shift-right: [w118] -> w108
              shift-left: dbl[] [] -> [w117]
              i -> [w131]
              stop <- w128 stop-if-true
              w123 = i32[] [1, 4] ("ActiveChannels")
              n180 = local read "Y(all)"() -> (w120:dbl[])
              n181 = Array Max & Min(array=w120) -> (max value=w119:dbl)  [unwired: 3 out]
              n182 = Build Array (concatenate)(w117, w119) -> (w118:dbl[])
              n183 = for {
                N: "channel on" -> [_]
                tunnel: w135 -> [w145]
                tunnel: [w144] -> w134
                tunnel: i8[] [1, 1] ("waveform") -> [w143] mode=indexing
                tunnel: w123 -> [w141] mode=indexing
                tunnel: [w140] -> w132 mode=indexing
                shift-right: [w142] -> w133
                shift-left: w126 -> [w146]
                tunnel: w127 -> [w137]
                tunnel: [w136] -> w124 mode=indexing
                i -> [w139]
                n184 = Equal To 0?(x=w139) -> (x = 0?=w138:bool)
                n185 = case shown="True" w138 {
                  tunnel: w146 -> [w165 w176]
                  tunnel: w145 -> [w164 _]
                  tunnel: [w163 w175] -> w144
                  tunnel: w143 -> [w162 w172]
                  tunnel: [w161 w171] -> w142
                  tunnel: w141 -> [w159 w170]
                  tunnel: [w160 w169] -> w140
                  tunnel: [w158 w166] -> w136
                  tunnel: w137 -> [w157 w168]
                  frame True {
                    n186 = call "rsscope Read Waveform.vi"("VISA resource name"=w157, "Waveform (1)"=w162, "Channel (1)"=w159, "Maximum Time (5000)"=w164, "error in (no error)"=w165) -> ("VISA resource name out"=w163:refnum<visa-resource-name>, "Waveform Array"=w154:dbl[], "Initial X"=w152:dbl, "X Increment"=w153:dbl, "error out"=w161:errorcluster)  [unwired: 6 in]
                    "Y(all)" <- w154
                    "X Increment" <- w153
                    "Initial X" <- w152
                    n187 = local read "X Increment"() -> (w148:dbl)
                    n188 = local read "Initial X"() -> (w147:dbl)
                    n189 = local read "T(all)"() -> (w151:dbl[])
                    n190 = local read "Y(all)"() -> (w150:dbl[])
                    n191 = Bundle("T(all)"=w151, "Y(all)"=w150, "X Increment"=w148, "Initial X"=w147) -> (→"output cluster":T4)  [unwired: 1 in]
                    n192 = call "data handle.vi"("Y"=w154, "X Increment (input)"=w153, "InitialX (input)"=w152) -> ("T"=w155:dbl[])  [unwired: 4 in, 3 out]
                    "T(all)" <- w155
                    n193 = Array Size(array=w154) -> (size(s)=w158:i32)
                    n194 = Bundle("Initial X"=w152, "X Increment"=w153, "Waveform Array"=w154) -> (w160:T17)  [unwired: 1 in]
                    n195 = Bundle("T"=w155, "Waveform Array"=w154) -> (→"waveform 3":cluster{"T":dbl[], "Waveform Array":dbl[]})  [unwired: 1 in]
                  }
                  frame False {
                    n196 = call "rsscope Fetch Waveform.vi"("Waveform (1)"=w172, "error in (no error)"=w176, "Channel (1)"=w170, "VISA resource name"=w168) -> ("error out"=w171:errorcluster, "Waveform Array"=w167:dbl[], "VISA resource name out"=w175:refnum<visa-resource-name>, "Initial X"=w173:dbl, "X Increment"=w174:dbl)  [unwired: 3 in]
                    n197 = Bundle("Initial X"=w173, "X Increment"=w174, "Waveform Array"=w167) -> (w169:T17)  [unwired: 1 in]
                    n198 = Array Size(array=w167) -> (size(s)=w166:i32)
                  }
                }
              }
              "Waveform" <- w132
              "Samples count" <- w124
              n199 = Unbundle By Name(w133) -> ("status"=w130:bool)
              n200 = Compound Arithmetic op=OR(w125, w130, "Stop") -> (w128:bool)
              "Acquisitions" <- w131
              "ActiveChannels" <- w123
            }
            "appended array" <- w108
          }
          event Timeout {
            n201 = event-data() -> ()  [unwired: 1 in, 2 out]
            n202 = local write "Tout"(-1 ("Tout")) -> ()
            n203 = for {
              N: 1 -> [_]
              tunnel: w178 -> [w186]
              shift-right: [w185] -> w181
              shift-left: w179 -> [w185]
              tunnel: [w184] -> _
              i -> [w182]
              n204 = call "Set Channel Enabled (CH1)"("instrument handle"=w186, "RepCap 'Channel' (CH1)"=w182, "Channel Enabled (OFF)"=TRUE) -> ("instrument handle out"=w184:refnum<visa-resource-name>)  [unwired: 11 in, 1 out]
            }
          }
          event "Exit": Value Change {
            n205 = event-data() -> ()  [unwired: 1 in, 1 out]
          }
        }
        n206 = property on="Stop" class="Bool"("Disabled"=u8 2) -> ()  [unwired: 2 in, 2 out]
        n207 = Unbundle By Name(w99) -> ("status"=w105:bool)
        n208 = Or(x=w105, y=w97) -> (x .or. y?=w106:bool)
      }
      n209 = while {
        tunnel: w89 -> [w243]
        tunnel: w88 -> [w242]
        tunnel: w83 -> [w241]
        shift-right: [w239] -> _
        shift-left: FALSE -> [w240]
        tunnel: [w238] -> w85
        tunnel: [w237] -> w84
        stop <- w245 stop-if-true
        n210 = property on="stop 2" class="Bool (strict)"() -> ("Value"=w236:bool)  [unwired: 2 in, 2 out]
        n211 = Dequeue Element(queue=w241, timeout in ms (-1)=50) -> (element=w247:T14, timed out?=w246:bool, error out=w250:errorcluster)  [unwired: 1 in, 1 out]
        n212 = Unbundle By Name(w250) -> ("status"=w249:bool)
        n213 = Or(x=w249, y=w236) -> (x .or. y?=w245:bool)
        n214 = case shown="False" w245 {
          tunnel: w242 -> [w257 w283]
          tunnel: w243 -> [w259 w284]
          tunnel: w247 -> [w253 _]
          tunnel: [w258 w284] -> w237
          tunnel: [w256 w283] -> w238
          tunnel: w246 -> [w255 _]
          tunnel: "Delay (ms)" -> [w254 _]
          tunnel: w240 -> [w252 w282]
          tunnel: [w251 w282] -> w239
          frame False {
            n215 = case shown="False" w255 {
              tunnel: w259 -> [w273 w281]
              tunnel: [w271 w281] -> w258
              tunnel: w257 -> [w272 w280]
              tunnel: [w270 w280] -> w256
              tunnel: w254 -> [w269 _]
              tunnel: w253 -> [w262 _]
              tunnel: w252 -> [w263 w279]
              tunnel: [w264 w279] -> w251
              frame False {
                w266 = u16 3 items=["MOVE", "HOME", "STOP", "Set Speed", "Info", "Set Zero"] ("Task")
                n216 = Unbundle By Name(w262) -> ("Task"=w261:u16)
                n217 = Equal?(x=w261, y=w266) -> (x = y?=w264:bool)
                n218 = Not(x=w264) -> (.not. x?=w265:bool)
                n219 = And(x=w263, y=w265) -> (x .and. y?=w260:bool)
                n220 = call "RS232 S&R 3.vi"("ReSetSPD"=w260, "error in"=w272, "Delay (ms)"=w269, "Stage Control"=w262, "VISA resource in"=w273) -> ("error out"=w270:errorcluster, "read"=w267:bool, "Cluster"=w268:T9, "VISA resource name out"=w271:refnum<visa-resource-name>)
                n221 = case shown="True" w267 {
                  tunnel: w268 -> [_ w278]
                  frame False {
                  }
                  frame True {
                    n222 = Unbundle By Name(w278) -> ("Current coordinates 2"=w276:cluster{"X":dbl, "Y":dbl, "Z":dbl})
                    "?" <- w276
                    n223 = Unbundle By Name(w278) -> ("Moving Time (Sec)"=→"Moving Time (Sec)":dbl)
                    n224 = feedback-in #1(w276) -> ()
                    n225 = feedback #1() -> (w275:cluster{"X":dbl, "Y":dbl, "Z":dbl})  [unwired: 1 in]
                    n226 = Equal?(x=w276, y=w275) -> (x = y?=→"Static":bool)
                    "Position Info" <- w278
                  }
                }
              }
              frame True {
              }
            }
          }
          frame True {
          }
        }
      }
      n227 = while {
        shift-right: [w194] -> w66
        shift-left: w63 -> [w196]
        shift-right: [w193] -> w65
        shift-left: w64 -> [w195]
        tunnel: w62 -> [w192]
        stop <- w191 stop-if-true
        n228 = case shown="True" "?" {
          tunnel: w196 -> [w197 w203]
          tunnel: w195 -> [w198 w202]
          tunnel: [w197 w201] -> w194
          tunnel: [w198 w200] -> w193
          tunnel: w192 -> [_ w199]
          frame False {
          }
          frame True {
            n229 = call <vilib>:"IMAQdx Grab.vi"("error in"=w202, "Image In"=w199, "Session In"=w203) -> ("error out"=w200:errorcluster, "Image Out"=w204:T2, "Session Out"=w201:T8)  [unwired: 1 in, 5 out]
            "Grab Image" <- w204
            n230 = case shown="True" "Get Image" {
              tunnel: w204 -> [_ w206]
              frame False {
              }
              frame True {
                "Snap Image" <- w206
              }
            }
          }
        }
        n231 = property on="stop 2" class="Bool (strict)"() -> ("Value"=w191:bool)  [unwired: 2 in, 2 out]
      }
      n232 = while {
        tunnel: w83 -> [w210]
        shift-right: [w208] -> _
        shift-left: 0 -> [w209]
        stop <- w207 stop-if-true
        w213 = 1000.0 ("value")
        w225 = u16 4 items=["MOVE", "HOME", "ZERO", "Set speed", "Info"] ("Ring")
        n233 = property on="Position to go" class="Clust (strict)"() -> ("Value"=w224:T7)  [unwired: 2 in, 2 out]
        n234 = Bundle("Ring"=w225, "Value"=w224) -> (w226:T18)  [unwired: 1 in]
        n235 = Enqueue Element(queue=w210, element=w226) -> (error out=w228:errorcluster)  [unwired: 2 in, 2 out]
        n236 = Unbundle By Name(w228) -> ("status"=w227:bool)
        n237 = property on="stop 2" class="Bool (strict)"() -> ("Value"=w229:bool)  [unwired: 2 in, 2 out]
        n238 = Or(x=w227, y=w229) -> (x .or. y?=w207:bool)
        n239 = case shown="False" w207 {
          frame False {
            n240 = Wait (ms)(milliseconds to wait="update period (ms)") -> ()  [unwired: 1 out]
          }
          frame True {
          }
        }
        n241 = property on="Moving Time (Sec)" class="DigNum (strict)"() -> ("Value"=w220:dbl)  [unwired: 2 in, 2 out]
        n242 = Tick Count (ms)() -> (millisecond timer value=w223:u32)
        n243 = First Call?() -> (First Call?: T/F=w222:bool)
        n244 = case shown="False" w222 {
          tunnel: w209 -> [w232 w233]
          tunnel: w223 -> [w231 w234]
          tunnel: [w231 w234] -> w208
          tunnel: [w230 w233] -> w221
          frame False {
            n245 = Subtract(x=w231, y=w232) -> (x-y=w230:u32)
          }
          frame True {
          }
        }
        n246 = Compound Arithmetic op=MULTIPLY(w213, w220) -> (w216:dbl)
        n247 = Not Equal To 0?(x=w216) -> (x != 0?=w212:bool)
        n248 = Subtract(x=w216, y=w221) -> (x-y=w218:dbl)
        n249 = Greater Than 0?(x=w218) -> (x > 0?=w217:bool)
        n250 = And(x=w217, y=w212) -> (x .and. y?=w211:bool)
        n251 = Select(t=w218, s=w211, f=0.0) -> (s? t:f=w214:dbl)
        n252 = Divide(x=w214, y=w213) -> (x/y=w215:dbl)
        n253 = property on="Moving Time (Sec)" class="DigNum (strict)"("Value"=w215) -> ()  [unwired: 2 in, 2 out]
      }
      n254 = call "rsscope Close.vi"("VISA resource name"=w51) -> ("error out"=w61:errorcluster)  [unwired: 10 in]
      n255 = call <vilib>:"Simple Error Handler.vi"("error in (no error)"=w61) -> ()  [unwired: 4 in, 5 out]
      n256 = call <vilib>:"IMAQdx Close Camera.vi"("error in"=w65, "Session In"=w66) -> ("error out"=w67:errorcluster)  [unwired: 9 out]
      n257 = call <vilib>:"Simple Error Handler.vi"("error in (no error)"=w67) -> ()  [unwired: 1 in, 8 out]
      n258 = VISA Close(VISA resource name=w77, error in (no error)=w76) -> ()  [unwired: 1 out]
      n259 = Release Queue(queue=w91, error in (no error)=w90) -> ()  [unwired: 1 in, 3 out]
      n260 = call "RS232 close.vi"("error in"=w85, "VISA resource name in"=w84) -> ("error out"=→"RS232 error":errorcluster)
    }
    frame #2 {
      n261 = property on="stop 2" class="Bool (strict)"("Value"=FALSE) -> ()  [unwired: 2 in, 2 out]
    }
  }
